vi "Error Handler Thread.vi"(7 "Data Path":path, 8 "error in (no error)":errorcluster, 10 "File Name":string, 11 "Cluster":T1={"Queue Array"=[], "Queue Element"={"state"="", "data"=variant}, "System Event"=refnum, "System Event RefNum"=refnum, "Queue List"=[], "LPCA COM"="", "Rotating"=FALSE, "PrecorAI"="", "T_0 Index"=0, "Bar Graph X"=[], "Channels"=[], "Active Indicies"=[], "Active Channels"=[], "Sample Frequency"=0.0, "Ibrake Sweep"=[], "RPM Sweep"=[], "Load Sweep"=[], "Step Height Sweep"=[], "Range Sweep"=[], "A Counter"=0, "B Counter"=0, "C Counter"=0, "#A"=0, "#B"=0, "#C"=0, "Current RPM"=0.0, "Current Ibrake"=0, "Current Range"=0, "Current Step Height"=0, "Load Bank"=enum."OFF", "Cfg Cntrls"=[], "T_Monitor Indices"=[], "Thermal Limit"=0, "Thermal Resume"=0, "Timer Reset"=FALSE, "Stop Time"=0.0, "Autotest"=FALSE, "Pulsed RPM Capture"=FALSE, "Get Sample"=FALSE, "Last State"="", "Reset Timeout"=FALSE, "Ctrl Refs"={"Test Details"=refnum, "Save Config"=refnum, "Load Config"=refnum, "Path"=refnum, "Snapshot"=refnum, "SS#"=refnum, "Ibrake"=refnum, "RPM Target"=refnum, "Spin"=refnum, "Load Bank"=refnum, "Start Test"=refnum, "Pause Test"=refnum, "Load Sweep"=refnum, "RPM Sweep"=refnum, "Ibrake Sweep"=refnum, "Filters"=refnum, "Sample Frequency"=refnum, "Data Setup"=refnum, "Pause"=refnum, "Stop Time"=refnum, "S Period"=refnum, "Range"=refnum, "Step Height"=refnum, "Step Height Sweep"=refnum, "Range Sweep"=refnum, "Available Tests"=refnum, "RPM Graph"=refnum, "RPM Knob"=refnum, "FanMode"=refnum, "Fan Mode LED Array"=refnum, "Thermal Equilibrium"=refnum, "Data Display"=refnum, "LPCA Error"=refnum, "LPCA Ramp"=refnum, "LPCA Range"=refnum, "LPCA Resistance"=refnum, "Analyze Read"=refnum, "Console Select"=refnum, "Sub Panel"=refnum}, "Pulse Waveform"={"t0"=timestamp(0 s since 1904-01-01), "dt"=1.0, "Y"=[]}, "Snapshot"={"Test Details"="test", "Version"="test", "Date"=timestamp(3493915594.3018084 s since 1904-01-01), "Selected Test"="man", "Snapshot Number"=0, "Time"=timestamp(3493915602.7292905 s since 1904-01-01), "Ibrake Setpoint"="1", "RPM Setpoint"="20", "Range Setpoint"="", "Step Height Setpoint"="", "Load Bank Setpoint"="15", "Measurement Headers"="a,b,c,1,2,3", "Measurements"="1,2,3,4,5,6,7,8", "A"=0, "B"=0, "C"=0, "Raw Data"=[], "Available Tests"=enum."Manual", "Ibrake List"="", "RPM List"="", "Load Bank List"="", "Range List"="", "Step Height List"="", "FanMode Setpoint"=enum."Auto"}, "Sample Period"=0.0, "OverTemp"=FALSE, "Available Tests"=enum."Manual", "FanMode"=enum."Auto", "Fan Mode LED Array"=[FALSE, TRUE, FALSE], "Thermal\nEquilibrium "=FALSE, "Equilibrium Stop"=FALSE, "AvgDegChg"=[]} {"Snapshot"."Time" format="%<%H:%M:%S>T"; "Snapshot"."Date" format="%<%m/%d/%Y>T"}) -> ()   [LabVIEW 2017]
uses:
  Source/Controls/Test TypeDef.ctl
  Queue References Array.ctl
  Queue Element.ctl
  Source/Controls/Load Bank.ctl
  Source/Controls/Available Tests.ctl
  Source/Console Sim/Controls/Console Select.ctl
  Source/Controls/Snapshot Typedef.ctl
  Source/Controls/FanMode.ctl
  <vilib>/Utility/sysdir.llb/System Directory Type.ctl
panel:
  out "Error Code Path":path
  in  "Custom Error Code Path":path=path "C:/programdata/crystaldetect/errorcodes.ini"
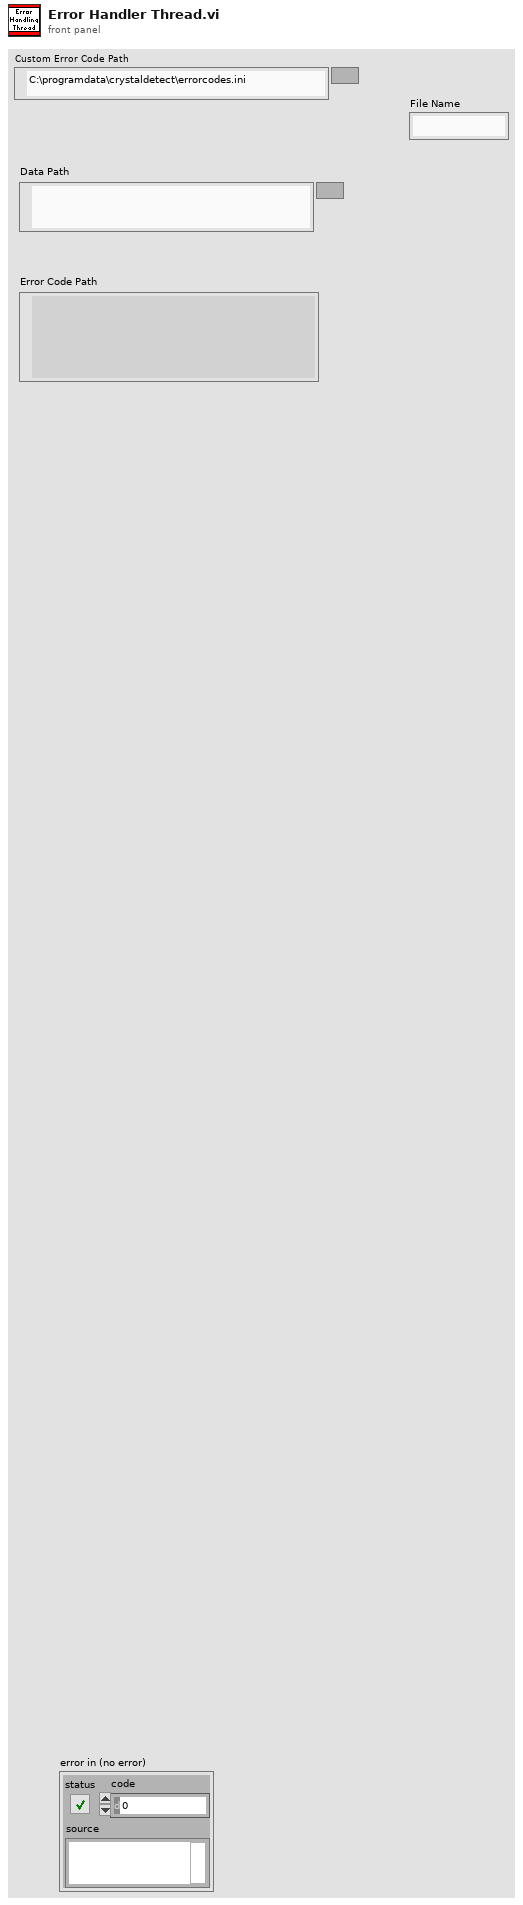
[diagram p1: front panel]
types:
  T1 = typedef "Test TypeDef.ctl" = cluster{"Queue Array":T2, "Queue Element":T3, "System Event":refnum<user-event>, "System Event RefNum":refnum<event-registration>, "Queue List":string[], "LPCA COM":refnum<visa-resource-name>, "Rotating":bool, "PrecorAI":refnum<k21>, "T_0 Index":i32, "Bar Graph X":i32[], "Channels":string[], "Active Indicies":i32[], "Active Channels":string[][], "Sample Frequency":dbl, "Ibrake Sweep":string[], "RPM Sweep":string[], "Load Sweep":string[], "Step Height Sweep":string[], "Range Sweep":string[], "A Counter":i32, "B Counter":i32, "C Counter":i32, "#A":i32, "#B":i32, "#C":i32, "Current RPM":dbl, "Current Ibrake":u32, "Current Range":u32, "Current Step Height":u32, "Load Bank":T4, "Cfg Cntrls":refnum<vi>[], "T_Monitor Indices":i32[], "Thermal Limit":i32, "Thermal Resume":i32, "Timer Reset":bool, "Stop Time":dbl, "Autotest":bool, "Pulsed RPM Capture":bool, "Get Sample":bool, "Last State":string, "Reset Timeout":bool, "Ctrl Refs":cluster{"Test Details":refnum<vi>, "Save Config":refnum<vi>, "Load Config":refnum<vi>, "Path":refnum<vi>, "Snapshot":refnum<vi>, "SS#":refnum<vi>, "Ibrake":refnum<vi>, "RPM Target":refnum<vi>, "Spin":refnum<vi>, "Load Bank":refnum<vi>, "Start Test":refnum<vi>, "Pause Test":refnum<vi>, "Load Sweep":refnum<vi>, "RPM Sweep":refnum<vi>, "Ibrake Sweep":refnum<vi>, "Filters":refnum<vi>, "Sample Frequency":refnum<vi>, "Data Setup":refnum<vi>, "Pause":refnum<vi>, "Stop Time":refnum<vi>, "S Period":refnum<vi>, "Range":refnum<vi>, "Step Height":refnum<vi>, "Step Height Sweep":refnum<vi>, "Range Sweep":refnum<vi>, "Available Tests":refnum<vi>, "RPM Graph":refnum<vi>, "RPM Knob":refnum<vi>, "FanMode":refnum<vi>, "Fan Mode LED Array":refnum<vi>, "Thermal Equilibrium":refnum<vi>, "Data Display":refnum<vi>, "LPCA Error":refnum<vi>, "LPCA Ramp":refnum<vi>, "LPCA Range":refnum<vi>, "LPCA Resistance":refnum<vi>, "Analyze Read":refnum<vi>, "Console Select":refnum<vi>, "Sub Panel":refnum<vi>}, "Pulse Waveform":waveform(dbl), "Snapshot":T5, "Sample Period":dbl, "OverTemp":bool, "Available Tests":T6, "FanMode":T7, "Fan Mode LED Array":bool[], "Thermal\nEquilibrium ":bool, "Equilibrium Stop":bool, "AvgDegChg":dbl[]}
  T2 = typedef "Queue References Array.ctl" = refnum<queue>[]
  T3 = typedef "Queue Element.ctl" = cluster{"state":string, "data":variant}
  T4 = typedef "Load Bank.ctl" = enum16{"OFF", "50", "25", "16.7", "12.5", "10.0", "8.3", "7.1", "6.3", "5.6", "5.0", "4.5", "4.2", "3.8", "3.6", "3.3", "3.1"}
  T5 = typedef "Snapshot Typedef.ctl" = cluster{"Test Details":string, "Version":string, "Date":timestamp, "Selected Test":string, "Snapshot Number":u16, "Time":timestamp, "Ibrake Setpoint":string, "RPM Setpoint":string, "Range Setpoint":string, "Step Height Setpoint":string, "Load Bank Setpoint":string, "Measurement Headers":string, "Measurements":string, "A":i32, "B":i32, "C":i32, "Raw Data":string[][], "Available Tests":T6, "Ibrake List":string, "RPM List":string, "Load Bank List":string, "Range List":string, "Step Height List":string, "FanMode Setpoint":T7}
  T6 = typedef "Available Tests.ctl" = enum16{"Manual", "EFX Brake Torque", "Generator Torque", "EFX Brake Thermal", "Generator Thermal", "Pulsed RPM", "AMT Brake Torque", "Bike Brake Torque", "AMT Brake Thermal", "Bike Brake Thermal"}
  T7 = typedef "FanMode.ctl" = enum16{"On", "Off", "Auto"}
  T8 = enum16{"open", "replace", "create", "open or create", "replace or create", "replace or create with confirmation"}
  T9 = enum16{"NULL", "Load Errors", "Add Errors", "Process Error"}
  T10 = typedef "System Directory Type.ctl" = i32
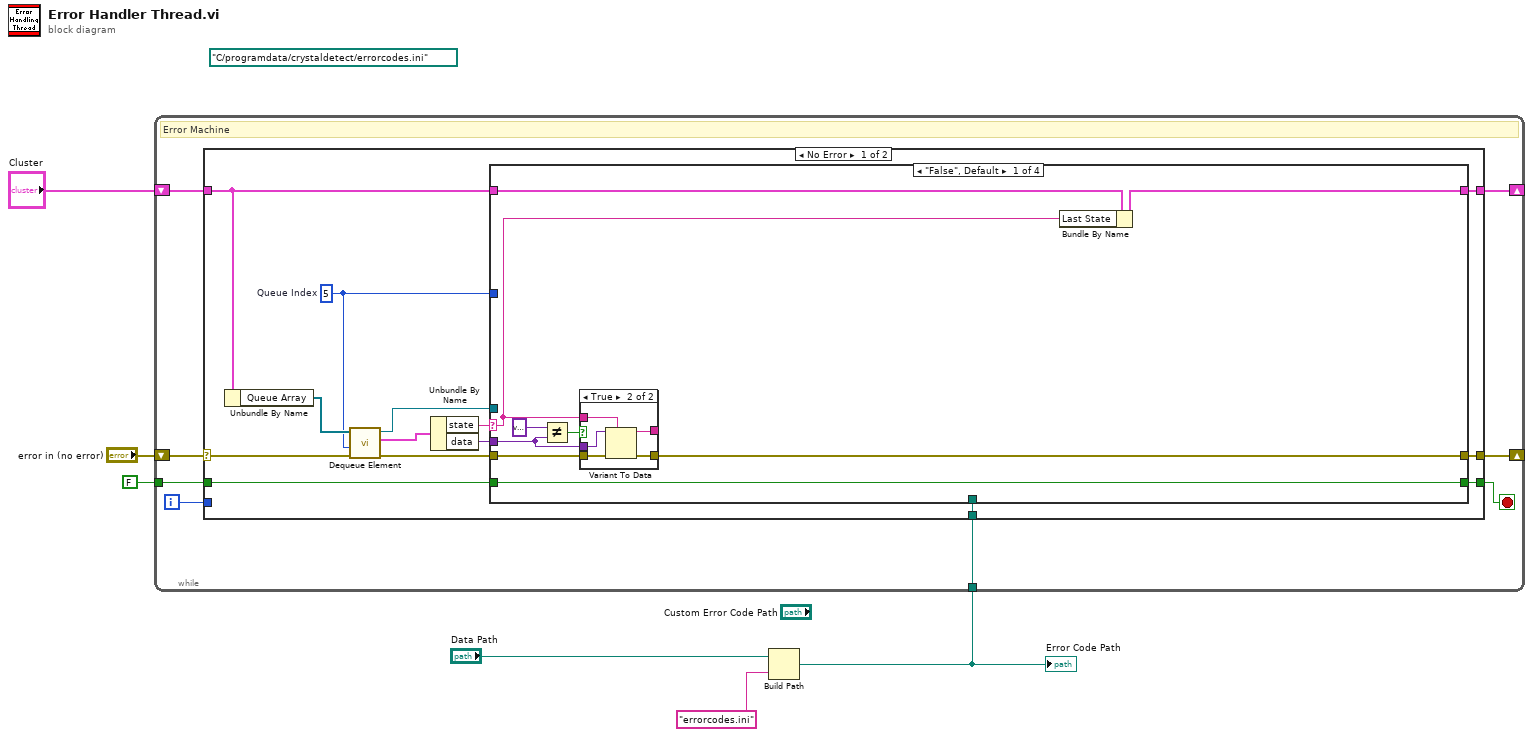
[diagram p0: block diagram]
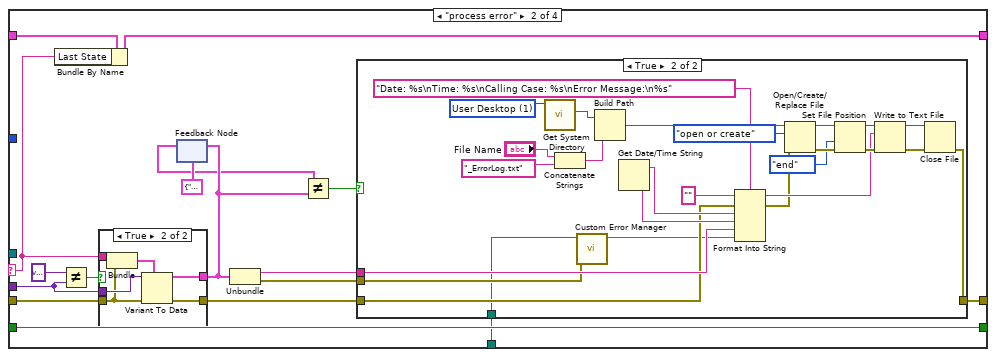
[diagram p3: hidden frame]
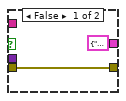
[diagram p5: hidden frame]
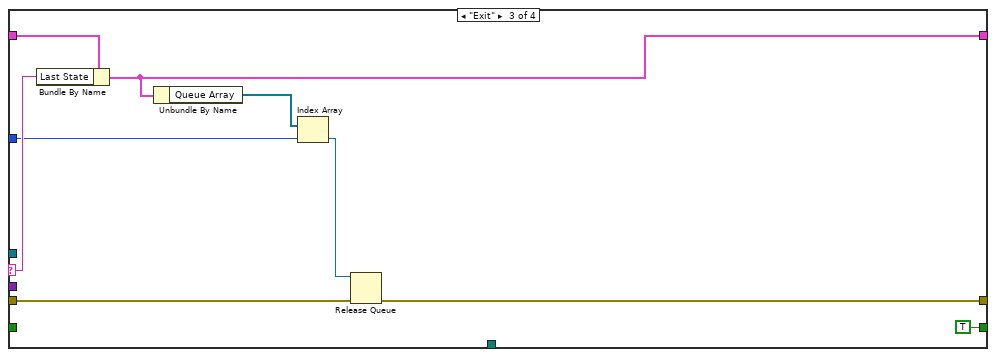
[diagram p6: hidden frame]
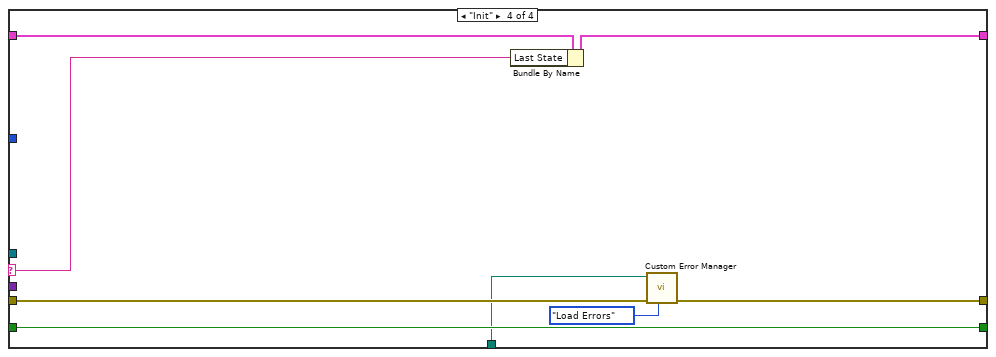
[diagram p7: hidden frame]
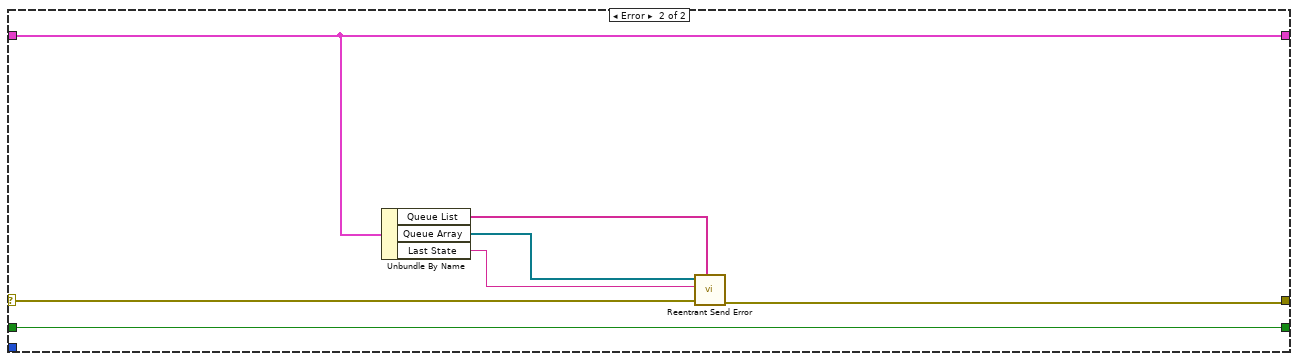
[diagram p8: hidden frame]
diagram:
  (unwired) path "C:/programdata/crystaldetect/errorcodes.ini" ("Custom Error Code Path")
  n1 = Build Path(base path="Data Path", name or relative path="errorcodes.ini") -> (appended path=w2:path)
  "Error Code Path" <- w2
  n2 = while "Error Machine" {
    shift-right: [w9] -> _
    shift-left: "Cluster" -> [w14]
    shift-right: [w10] -> _
    shift-left: "error in (no error)" -> [w11]
    tunnel: FALSE ("Boolean") -> [w13]
    tunnel: w2 -> [w7]
    i -> [w8]
    stop <- w12 stop-if-true
    # "Error Machine"
    n3 = case shown="No Error" w11 {
      selector: w11 -> [w20 w119]
      tunnel: w14 -> [w24 w117]
      tunnel: w13 -> [w26 w120]
      tunnel: [w27 w120] -> w12
      tunnel: [w28 w118] -> w10
      tunnel: [w25 w117] -> w9
      tunnel: w8 -> [_ _]
      tunnel: w7 -> [w15 _]
      frame No Error {
        w16 = 5  # Queue Index
        n4 = Unbundle By Name(w24) -> ("Queue Array"=w21:T2)
        n5 = call "Dequeue Element.vi"("error in (no error)"=w20, "index"=w16, "Queue Array"=w21) -> ("error out"=w19:errorcluster, "Queue Element"=w17:T3, "Queue Out"=w18:refnum<queue>)  [unwired: 6 in]
        n6 = Unbundle By Name(w17) -> ("state"=w23:string, "data"=w22:variant)
        n7 = case shown="\"False\", Default" w23 {
          selector: w23 -> [w31 w55 w103 w110]
          tunnel: [w34 w51 w105 w109] -> w28
          tunnel: w19 -> [w35 w59 w102 w107]
          tunnel: [w37 w61 TRUE ("Boolean") w113] -> w27
          tunnel: w26 -> [w37 w61 _ w113]
          tunnel: [w29 w56 w100 w111] -> w25
          tunnel: w24 -> [w30 w46 w104 w112]
          tunnel: w22 -> [w32 w57 _ _]
          tunnel: w18 -> [_ _ _ _]
          tunnel: w16 -> [_ _ w98 _]
          tunnel: w15 -> [_ w45 _ w106]
          frame "False", Default {
            n8 = Not Equal?(x=variant, y=w32) -> (x != y?=w33:bool)
            n9 = case shown="True" w33 {
              tunnel: w35 -> [w39 w44]
              tunnel: [w39 w43] -> w34
              tunnel: w31 -> [w38 w42]
              tunnel: w32 -> [_ w41]
              tunnel: [w38 w40] -> _
              frame False {
              }
              frame True {
                n10 = Variant To Data(error in=w44, type=w42, Variant=w41) -> (data=w40:string, error out=w43:errorcluster)
              }
            }
            n11 = Bundle By Name(cluster=w30, "Last State"=w31) -> (w29:T1)
          }
          frame "process error" {
            n12 = Bundle By Name(cluster=w46, "Last State"=w55) -> (w56:T1)
            n13 = Not Equal?(x=variant, y=w57) -> (x != y?=w58:bool)
            n14 = case shown="True" w58 {
              tunnel: w59 -> [w90 w92]
              tunnel: [w90 w96] -> w52
              tunnel: w57 -> [_ w95]
              tunnel: [cluster{string, "error IO":errorcluster} {"", "error IO"={"status"=FALSE, "code"=0, "source"=""}} w94] -> w49
              tunnel: w55 -> [_ w93]
              frame False {
              }
              frame True {
                n15 = Bundle(w93, "error out"=w92) -> (w91:cluster{string, "error out":errorcluster})  [unwired: 1 in]
                n16 = Variant To Data(error in=w92, type=w91, Variant=w95) -> (data=w94:cluster{string, "error out":errorcluster}, error out=w96:errorcluster)
              }
            }
            n17 = feedback #1(cluster{string, "error IO":errorcluster} {"", "error IO"={"status"=FALSE, "code"=0, "source"=""}} ("cluster")) -> (w48:cluster{string, "error IO":errorcluster})
            n18 = feedback-in #1(w49) -> ()
            n19 = Unbundle(w49) -> (w53:string, "error out"=w54:errorcluster)
            n20 = Not Equal?(x=w48, y=w49) -> (x != y?=w47:bool)
            n21 = case shown="True" w47 {
              tunnel: w54 -> [_ w65]
              tunnel: w53 -> [_ w82]
              tunnel: w52 -> [w62 w69]
              tunnel: [w62 w68] -> w51
              tunnel: w45 -> [_ w63]
              frame False {
              }
              frame True {
                w88 = T10 1 items=["User Home"=0, "User Desktop"=1, "User Documents"=2, "User Application Data"=3, "User Preferences"=4, "User Temporary"=5, "Public Documents"=6, "Public Application Data"=7, "Public Preferences"=8, "Public Cache"=13, "System Core Libraries"=9, "System Installed Libraries"=10, "Application Files"=11, "Boot Volume Root"=12] ("system directory type")
                n22 = call <vilib>:"Get System Directory.vi"("system directory type"=w88) -> ("system directory"=w87:path)  [unwired: 10 in]
                n23 = Concatenate Strings("File Name", "_ErrorLog.txt" ("name or relative path")) -> (w67:string)
                n24 = call "Custom Error Manager.vi"("error in (no error)"=w65, "Custom Error Code Path"=w63) -> ("Error String"=w64:string)  [unwired: 8 in, 1 out]
                n25 = Build Path(base path=w87, name or relative path=w67) -> (appended path=w80:path)
                n26 = Get Date/Time String() -> (date string=w84:string, time string=w83:string)  [unwired: 3 in]
                n27 = Format Into String(format string="Date: %s\nTime: %s\nCalling Case: %s\nError Message:\n%s", initial string="", error in=w69, w84, w83, w82, w64) -> (resulting string=w71:string, error out=w70:errorcluster)
                n28 = Open/Create/Replace File(file path (use dialog)=w80, error in=w70, operation (0:open)=T8."open or create") -> (refnum out=w77:refnum<file>, error out=w78:errorcluster)  [unwired: 3 in, 1 out]
                n29 = Set File Position(refnum=w77, from (0:start)=enum16{"start", "end", "current"}."end", error in=w78) -> (refnum out=w73:refnum<file>, error out=w76:errorcluster)  [unwired: 1 in]
                n30 = Write to Text File(file (use dialog)=w73, text=w71, error in=w76) -> (refnum out=w74:refnum<file>, error out=w75:errorcluster)  [unwired: 1 in, 1 out]
                n31 = Close File(refnum=w74, error in=w75) -> (error out=w68:errorcluster)  [unwired: 1 out]
              }
            }
          }
          frame "Exit" {
            n32 = Bundle By Name(cluster=w104, "Last State"=w103) -> (w100:T1)
            n33 = Unbundle By Name(w100) -> ("Queue Array"=w99:T2)
            n34 = Index Array(array=w99, index=w98) -> (element=w97:refnum<queue>)
            n35 = Release Queue(queue=w97, error in (no error)=w102) -> (error out=w105:errorcluster)  [unwired: 1 in, 2 out]
          }
          frame "Init" {
            n36 = Bundle By Name(cluster=w112, "Last State"=w110) -> (w111:T1)
            n37 = call "Custom Error Manager.vi"("Mode"=T9."Load Errors", "error in (no error)"=w107, "Custom Error Code Path"=w106) -> ("error out"=w109:errorcluster)  [unwired: 7 in, 1 out]
          }
        }
      }
      frame Error {
        n38 = Unbundle By Name(w117) -> ("Queue List"=w114:string[], "Queue Array"=w115:T2, "Last State"=w116:string)
        n39 = call "Reentrant Send Error.vi"("Queue Names"=w114, "error in (no error)"=w119, "Last State"=w116, "Queues"=w115) -> ("error out"=w118:errorcluster)  [unwired: 7 in]
      }
    }
  }
